vi "Read Attributes.vi"(11 "Direct Message Msg":refnum<class "Direct Message Msg.lvclass">) -> (2 "Payload":cluster{"Message":T1})   [LabVIEW 2014, in "Chat Window UI Controller.lvlib" / "Direct Message Msg.lvclass"]
uses:
  Direct Message Msg.lvclass
  Controls/Message Control.ctl
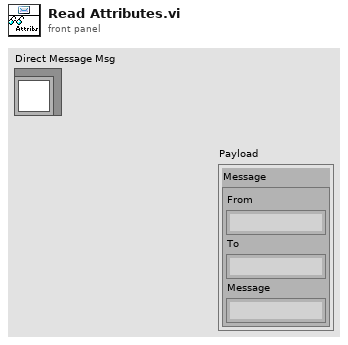
[diagram p1: front panel]
types:
  T1 = typedef "Message Control.ctl" = cluster{"From":string, "To":string, "Message":string}
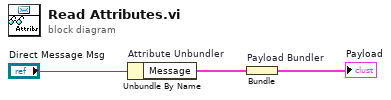
[diagram p0: block diagram]
diagram:
  n1 = Unbundle By Name "Attribute Unbundler"("Direct Message Msg") -> ("Message"=w1:T1)
  n2 = Bundle "Payload Bundler"("Message"=w1) -> (→"Payload":cluster{"Message":T1})  [unwired: 1 in]
